vi "测量数据区.vi"(11 "数组":u16[](array[numeric]) format="%04xH") -> (3 "测量数据区":T1 {"单位" items=["ug/L", "mg/L", "ppm", "mg/m3", "cm", "ppb", "ug/m3", "%", "nmol/mol", "umol/mol", "MPN/L", "MPN/100ml", "ng/m3", "NTU", "无量纲", "ms/cm", "us/cm", "℃", "mV", "万个/L"]})   [LabVIEW 2016, in "斯坦道仪器.lvlib"]
panel:
  # "共占用104 WORD"
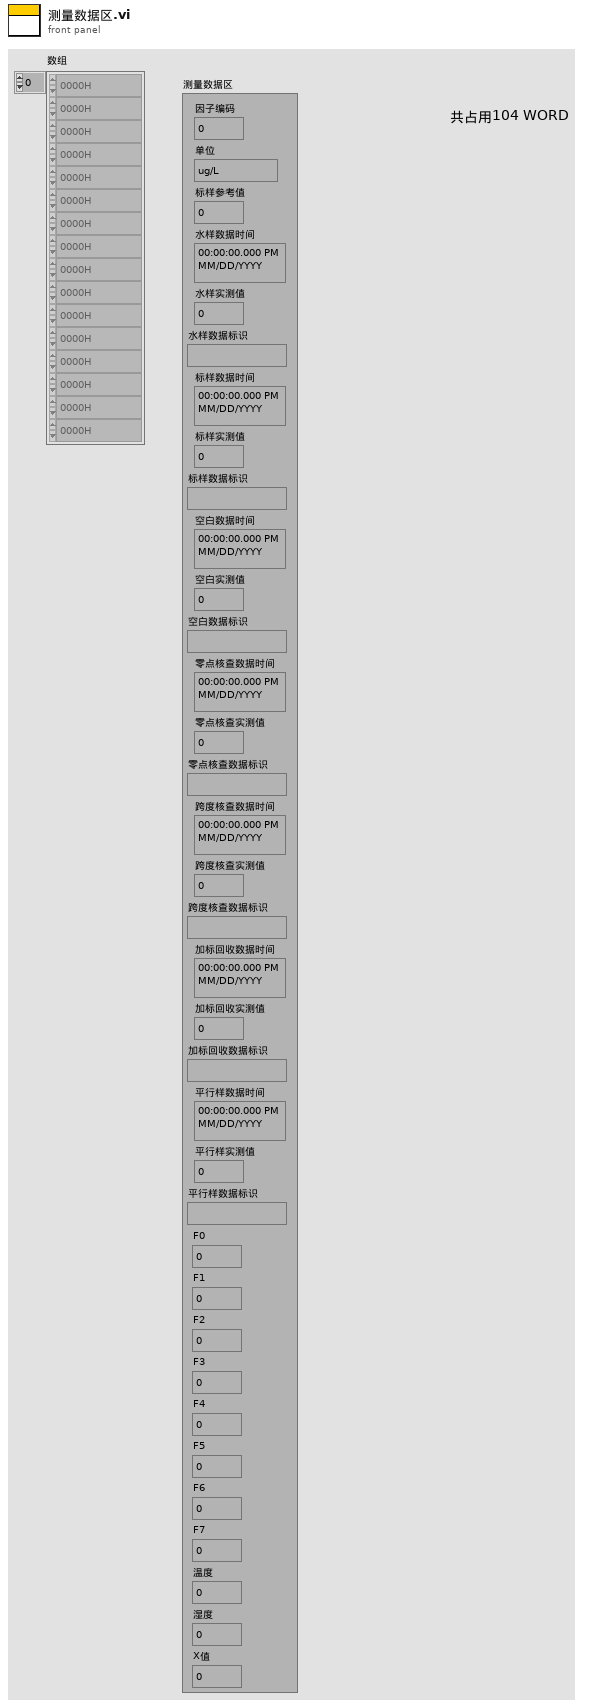
[diagram p1: front panel]
types:
  T1 = cluster{"因子编码":u32, "单位":u16, "标样参考值":sgl, "水样数据时间":timestamp, "水样实测值":sgl, "水样数据标识":string, "标样数据时间":timestamp, "标样实测值":sgl, "标样数据标识":string, "空白数据时间":timestamp, "空白实测值":sgl, "空白数据标识":string, "零点核查数据时间":timestamp, "零点核查实测值":sgl, "零点核查数据标识":string, "跨度核查数据时间":timestamp, "跨度核查实测值":sgl, "跨度核查数据标识":string, "加标回收数据时间":timestamp, "加标回收实测值":sgl, "加标回收数据标识":string, "平行样数据时间":timestamp, "平行样实测值":sgl, "平行样数据标识":string, "F0":sgl, "F1":sgl, "F2":sgl, "F3":sgl, "F4":sgl, "F5":sgl, "F6":sgl, "F7":sgl, "温度":sgl, "湿度":sgl, "X值":sgl}
  T2 = cluster{"DWORD":i32, "WORD":u16, "FLOAT":sgl, "time stamp":timestamp, "数值":sgl, "string":string, "time stamp":timestamp, "数值":sgl, "string":string, "time stamp":timestamp, "数值":sgl, "string":string, "time stamp":timestamp, "数值":sgl, "string":string, "time stamp":timestamp, "数值":sgl, "string":string, "time stamp":timestamp, "数值":sgl, "string":string, "time stamp":timestamp, "数值":sgl, "string":string, "FLOAT":sgl, "FLOAT":sgl, "FLOAT":sgl, "FLOAT":sgl, "FLOAT":sgl, "FLOAT":sgl, "FLOAT":sgl, "FLOAT":sgl, "FLOAT":sgl, "FLOAT":sgl, "FLOAT":sgl}
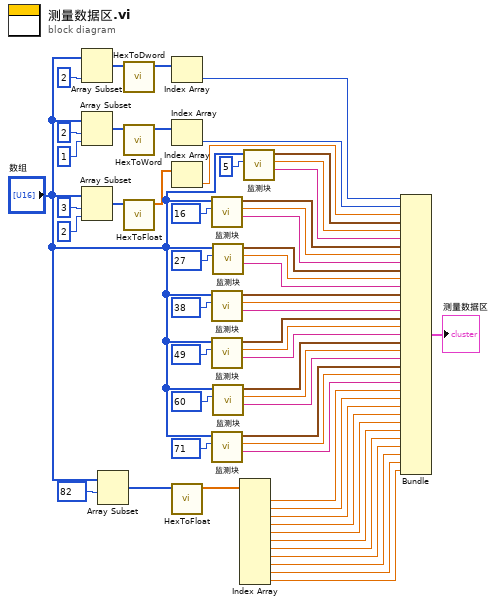
[diagram p0: block diagram]
diagram:
  n1 = Array Subset(array="数组", length=2 ("长度")) -> (w58:u16[])  [unwired: 1 in]
  n2 = Array Subset(array="数组", index=2 ("索引"), length=1 ("长度")) -> (w53:u16[])
  n3 = Array Subset(array="数组", index=3 ("索引"), length=2 ("长度")) -> (w48:u16[])
  n4 = Array Subset(array="数组", index=82 ("索引")) -> (w13:u16[])  [unwired: 1 in]
  n5 = call "HexToDword.vi"("数组"=w58) -> ("DWORD"=w56:i32[])  [unwired: 10 in]
  n6 = call "HexToWord.vi"("数组"=w53) -> ("WORD"=w52:u16[])  [unwired: 10 in]
  n7 = call "HexToFloat.vi"("数组"=w48) -> ("FLOAT"=w47:sgl[])  [unwired: 10 in]
  n8 = Index Array(array=w56) -> (element=w17:i32)  [unwired: 1 in]
  n9 = Index Array(array=w52) -> (element=w51:u16)  [unwired: 1 in]
  n10 = Index Array(array=w47) -> (element=w46:sgl)  [unwired: 1 in]
  n11 = call "HexToFloat.vi"("数组"=w13) -> ("FLOAT"=w12:sgl[])  [unwired: 10 in]
  n12 = call "监测块.vi"("索引"=16, "数组"="数组") -> ("string"=w38:string, "数值"=w39:sgl, "time stamp"=w40:timestamp)  [unwired: 7 in]
  n13 = call "监测块.vi"("索引"=38, "数组"="数组") -> ("string"=w30:string, "数值"=w31:sgl, "time stamp"=w32:timestamp)  [unwired: 7 in]
  n14 = call "监测块.vi"("索引"=49, "数组"="数组") -> ("string"=w26:string, "数值"=w27:sgl, "time stamp"=w28:timestamp)  [unwired: 7 in]
  n15 = call "监测块.vi"("索引"=71, "数组"="数组") -> ("string"=w18:string, "数值"=w19:sgl, "time stamp"=w20:timestamp)  [unwired: 7 in]
  n16 = call "监测块.vi"("索引"=27, "数组"="数组") -> ("string"=w34:string, "数值"=w35:sgl, "time stamp"=w36:timestamp)  [unwired: 7 in]
  n17 = call "监测块.vi"("索引"=60, "数组"="数组") -> ("string"=w22:string, "数值"=w23:sgl, "time stamp"=w24:timestamp)  [unwired: 7 in]
  n18 = Index Array(array=w12) -> (element #1=w11:sgl, element #2=w10:sgl, element #3=w9:sgl, element #4=w8:sgl, element #5=w7:sgl, element #6=w6:sgl, element #7=w5:sgl, element #8=w4:sgl, element #9=w3:sgl, element #10=w2:sgl, element #11=w1:sgl)  [unwired: 11 in]
  n19 = call "监测块.vi"("索引"=5, "数组"="数组") -> ("string"=w43:string, "数值"=w44:sgl, "time stamp"=w45:timestamp)  [unwired: 7 in]
  n20 = Bundle("DWORD"=w17, "WORD"=w51, "FLOAT"=w46, "time stamp"=w45, "数值"=w44, "string"=w43, "time stamp"=w40, "数值"=w39, "string"=w38, "time stamp"=w36, "数值"=w35, "string"=w34, "time stamp"=w32, "数值"=w31, "string"=w30, "time stamp"=w28, "数值"=w27, "string"=w26, "time stamp"=w24, "数值"=w23, "string"=w22, "time stamp"=w20, "数值"=w19, "string"=w18, "FLOAT"=w11, "FLOAT"=w10, "FLOAT"=w9, "FLOAT"=w8, "FLOAT"=w7, "FLOAT"=w6, "FLOAT"=w5, "FLOAT"=w4, "FLOAT"=w3, "FLOAT"=w2, "FLOAT"=w1) -> (→"测量数据区":T2)  [unwired: 1 in]
